vi "Write Characters to File - With Error in and Error Out - __jki_lib_file -- VI Tester.vi"(0 "file path (dialog if empty)":path, 5 "character string":string, 7 "append to file? (new file:F)":bool, 9 "prompt":string="Choose file to write.", 11 "error in (no error)":errorcluster, 12 "convert eol? (no:F)":bool) -> (4 "new file path (Not A Path if cancelled)":path, 15 "error out":errorcluster)   [LabVIEW 2011]
panel:
  # "Copyright © 2006 James Kring, Inc. All rights reserved.\n\nAuthor: Philippe Guerit [philippe.guerit@jameskring.com]\n             [alternate email: PJM_LabVIEW@yahoo.com]\n\nThis library is provided \"AS IS\" ,WITHOUT WARRANTIES OR \nCONDITIONS OF ANY KIND, either express or implied.\n\nJames Kring, Inc. -- http://www.jameskring.com"
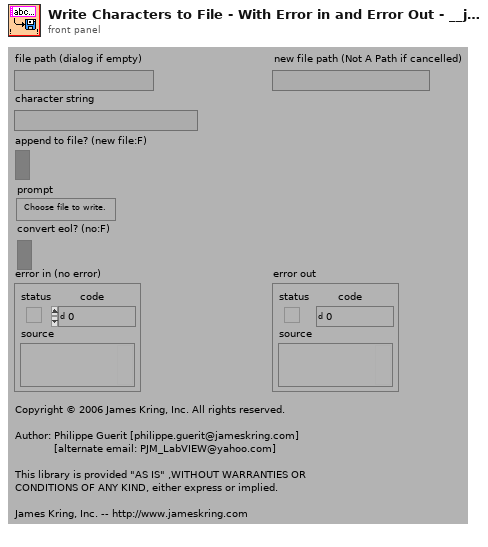
[diagram p1: front panel]
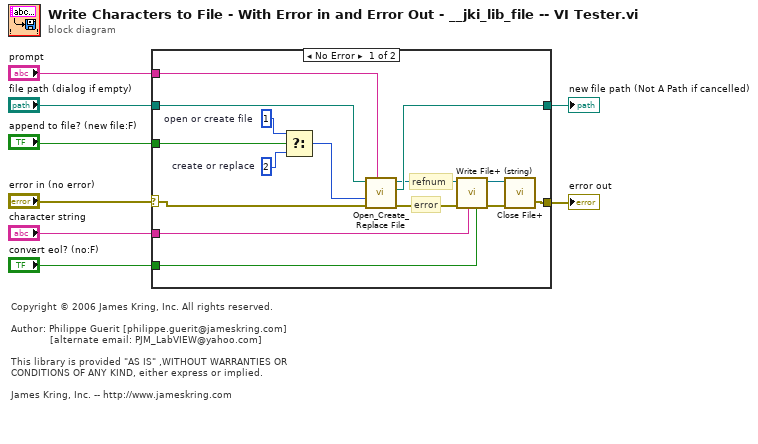
[diagram p0: block diagram]
diagram:
  # "Copyright © 2006 James Kring, Inc. All rights reserved.\n\nAuthor: Philippe Guerit [philippe.guerit@jameskring.com]\n             [alternate email: PJM_LabVIEW@yahoo.com]\n\nThis library is provided \"AS IS\" ,WITHOUT WARRANTIES OR \nCONDITIONS OF ANY KIND, either express or implied.\n\nJames Kring, Inc. -- http://www.jameskring.com"
  n1 = case shown="No Error" "error in (no error)" {
    selector: "error in (no error)" -> [w9 w25]
    tunnel: "prompt" -> [w23 _]
    tunnel: "convert eol? (no:F)" -> [w22 _]
    tunnel: [w21 w24] -> w6
    tunnel: "character string" -> [w18 _]
    tunnel: "append to file? (new file:F)" -> [w17 _]
    tunnel: "file path (dialog if empty)" -> [w11 w24]
    tunnel: [w10 w25] -> w2
    frame No Error {
      w19 = i16 2  # create or replace
      w16 = i16 1  # open or create file
      # "error"
      # "refnum"
      n2 = Select(t=w16, s=w17, f=w19) -> (s? t:f=w15:i16)
      n3 = call <vilib>:"Open_Create_Replace File.vi"("prompt"=w23, "error in (no error)"=w9, "function (open:0)"=w15, "file path"=w11) -> ("error out"=w12:errorcluster, "new file path"=w21:path, "refnum"=w20:refnum<file>)  [unwired: 4 in, 1 out]
      n4 = call <vilib>:"Write File+ (string).vi"("convert eol? (no:F)"=w22, "string"=w18, "error in (no error)"=w12, "refnum"=w20) -> ("error out"=w13:errorcluster, "dup refnum"=w14:refnum<file>)  [unwired: 3 in, 1 out]
      n5 = call <vilib>:"Close File+.vi"("error in (no error)"=w13, "refnum"=w14) -> ("error out"=w10:errorcluster)  [unwired: 3 in, 2 out]
    }
    frame Error {
    }
  }
  "error out" <- w2
  "new file path (Not A Path if cancelled)" <- w6
